vi "rs3_RGB_to_Picture3.vi"(0 "RGB array":u8[](array[numeric]), 2 "Color(T)/Greyscale(F)":bool, 5 "RGB  X, width":i32, 7 "RGB Y, height":i32, 9 "AWB":bool, 11 "error in (no error)":errorcluster, 12 "White Balance":cluster{"Red":dbl, "Green":dbl, "Blue":dbl}={"Red"=1.0, "Green"=1.0, "Blue"=1.0} {"Blue" format="%_3g"; "Green" format="%_3g"; "Red" format="%_3g"}, 14 "White Balance":bool) -> (6 "new picture":picture, 15 "error out":errorcluster)   [LabVIEW 2017, in "libRealSense3.lvlib"]
doc: "This converts an 1D input array into a 2D picture, and applies some white balance correction if requested."
uses:
  <vilib>/addons/RealSense/libRealSense3.lvlib
  <vilib>/Analysis/baseanly.llb/Mean (DBL).vi
  <vilib>/Analysis/NI_AALBase.lvlib
panel:
  # "RS3 RGB to Picture"
  # "(C) Intel Corp. 2017,  AGJ"
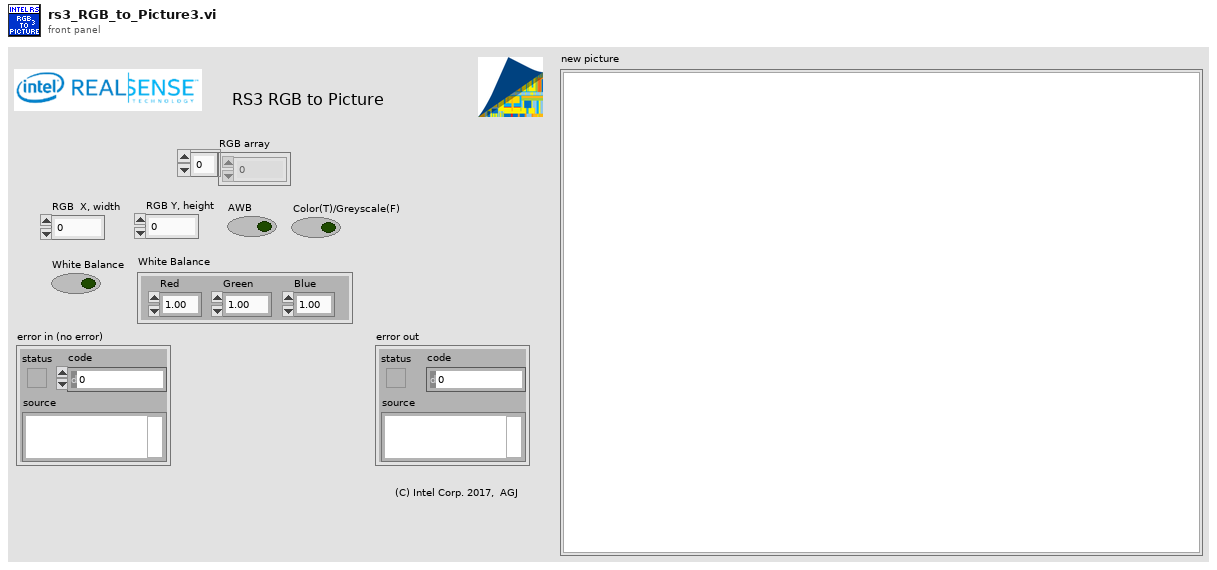
[diagram p1: front panel]
types:
  T1 = typedef "imagedata.ctl" = cluster{"image type":i32, "image depth":i32, "image":u8[], "mask":u8[], "colors":u32[], "Rectangle":cluster{"left":i16, "top":i16, "right":i16, "bottom":i16}}
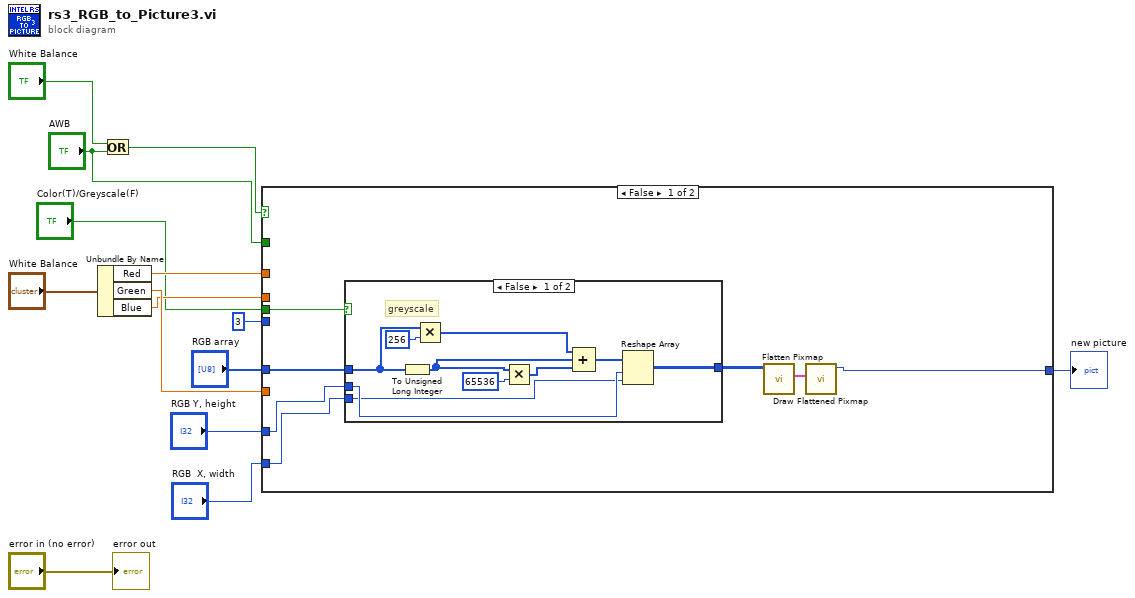
[diagram p0: block diagram]
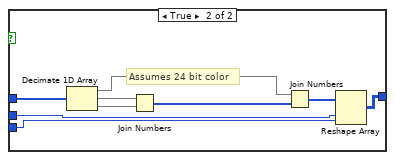
[diagram p2: hidden frame]
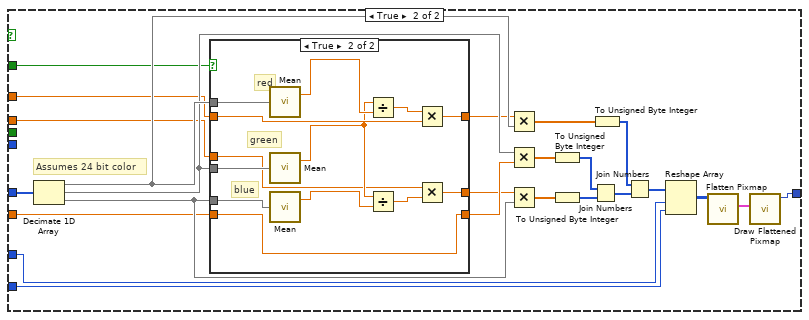
[diagram p3: hidden frame]
diagram:
  n1 = Unbundle By Name("White Balance") -> ("Red"=w9:dbl, "Green"=w8:dbl, "Blue"=w7:dbl)
  n2 = Or(x="White Balance", y="AWB") -> (x .or. y?=w2:bool)
  n3 = case shown="False" w2 {
    tunnel: [w21 w52] -> w14
    tunnel: "RGB array" -> [w20 w60]
    tunnel: "RGB Y, height" -> [w19 w51]
    tunnel: "RGB  X, width" -> [w18 w59]
    tunnel: 3 ("# of bytes/number") -> [_ _]
    tunnel: w9 -> [_ w46]
    tunnel: w8 -> [_ w44]
    tunnel: w7 -> [_ w43]
    tunnel: "AWB" -> [_ w41]
    tunnel: "Color(T)/Greyscale(F)" -> [w17 _]
    frame False {
      n4 = case shown="False" w17 {
        tunnel: [w29 w39] -> w16
        tunnel: w20 -> [w25 w37]
        tunnel: w19 -> [w31 w36]
        tunnel: w18 -> [w30 w35]
        frame False {
          # "greyscale"
          n5 = To Unsigned Long Integer(number=w25) -> (unsigned 32bit integer=w22:u32[])
          n6 = Multiply(x=w25, y=u32 256) -> (x*y=w26:u32[])
          n7 = Multiply(x=w22, y=u32 65536) -> (x*y=w24:u32[])
          n8 = Compound Arithmetic op=ADD(w26, w22, w24) -> (w23:u32[])
          n9 = Reshape Array(w23, w31, w30) -> (w29:u32[][])
        }
        frame True {
          # "Assumes 24 bit color"
          n10 = Decimate 1D Array(w37) -> (w34:u8[], w33:u8[], w32:u8[])
          n11 = Join Numbers(hi=w33, lo=w32) -> ((hi.lo)=w40:u16[])
          n12 = Join Numbers(hi=w34, lo=w40) -> ((hi.lo)=w38:u32[])
          n13 = Reshape Array(w38, w36, w35) -> (w39:u32[][])
        }
      }
      n14 = call <vilib>:"Flatten Pixmap.vi"("24-bit pixmap"=w16) -> ("image data"=w15:T1)  [unwired: 10 in]
      n15 = call <vilib>:"Draw Flattened Pixmap.vi"("image data"=w15) -> ("new picture"=w21:picture)  [unwired: 8 in]
    }
    frame True {
      # "Assumes 24 bit color"
      n16 = Decimate 1D Array(w60) -> (w50:u8[], w49:u8[], w48:u8[])
      n17 = case shown="True" w41 {
        tunnel: w50 -> [_ w80]
        tunnel: w49 -> [_ w79]
        tunnel: w48 -> [_ w78]
        tunnel: [w67 w73] -> w47
        tunnel: w46 -> [w67 w74]
        tunnel: [w66 w68] -> w45
        tunnel: w44 -> [w66 w68]
        tunnel: w43 -> [w65 w70]
        tunnel: [w65 w69] -> w42
        frame False {
        }
        frame True {
          # "blue"
          # "green"
          # "red"
          n18 = call-poly <vilib>:"Mean.vi"("X"=w80) -> ("mean"=w77:dbl)  [unwired: 1 out]
          n19 = call-poly <vilib>:"Mean.vi"("X"=w79) -> ("mean"=w72:dbl)  [unwired: 1 out]
          n20 = call-poly <vilib>:"Mean.vi"("X"=w78) -> ("mean"=w76:dbl)  [unwired: 1 out]
          n21 = Divide(x=w72, y=w77) -> (x/y=w75:dbl)
          n22 = Divide(x=w72, y=w76) -> (x/y=w71:dbl)
          n23 = Multiply(x=w75, y=w74) -> (x*y=w73:dbl)
          n24 = Multiply(x=w70, y=w71) -> (x*y=w69:dbl)
        }
      }
      n25 = Multiply(x=w47, y=w50) -> (x*y=w58:dbl[])
      n26 = Multiply(x=w49, y=w45) -> (x*y=w54:dbl[])
      n27 = Multiply(x=w42, y=w48) -> (x*y=w55:dbl[])
      n28 = To Unsigned Byte Integer(number=w54) -> (unsigned 8bit integer=w56:u8[])
      n29 = To Unsigned Byte Integer(number=w55) -> (unsigned 8bit integer=w53:u8[])
      n30 = Join Numbers(hi=w56, lo=w53) -> ((hi.lo)=w64:u16[])
      n31 = To Unsigned Byte Integer(number=w58) -> (unsigned 8bit integer=w57:u8[])
      n32 = Join Numbers(hi=w57, lo=w64) -> ((hi.lo)=w61:u32[])
      n33 = Reshape Array(w61, w51, w59) -> (w63:u32[][])
      n34 = call <vilib>:"Flatten Pixmap.vi"("24-bit pixmap"=w63) -> ("image data"=w62:T1)  [unwired: 10 in]
      n35 = call <vilib>:"Draw Flattened Pixmap.vi"("image data"=w62) -> ("new picture"=w52:picture)  [unwired: 8 in]
    }
  }
  "new picture" <- w14
  "error out" <- "error in (no error)"
